vi "SettingsDialog.vi"(8 "error in (no error)":errorcluster, 11 "ProgramSettings in":refnum<class "ProgramSettings.lvclass">) -> (0 "error out":errorcluster, 3 "ProgramSettings out":refnum<class "ProgramSettings.lvclass">)   [LabVIEW 2019, in "ProgramSettings.lvclass"]
uses:
  ProgramSettings.lvclass
  ProgramSettings.lvclass/ProgramSettings.ctl
panel:
  in  "Settings":T1={"Serial Port for strømforsyning"="COM12"}
  in  "Cancel":bool
  in  "OK":bool
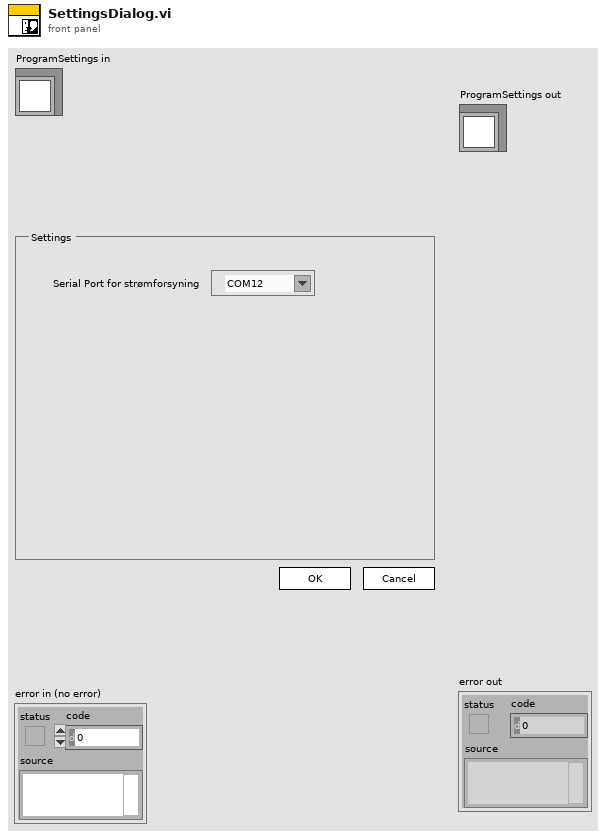
[diagram p1: front panel]
types:
  T1 = cluster{"Serial Port for strømforsyning":refnum<visa-resource-name>}
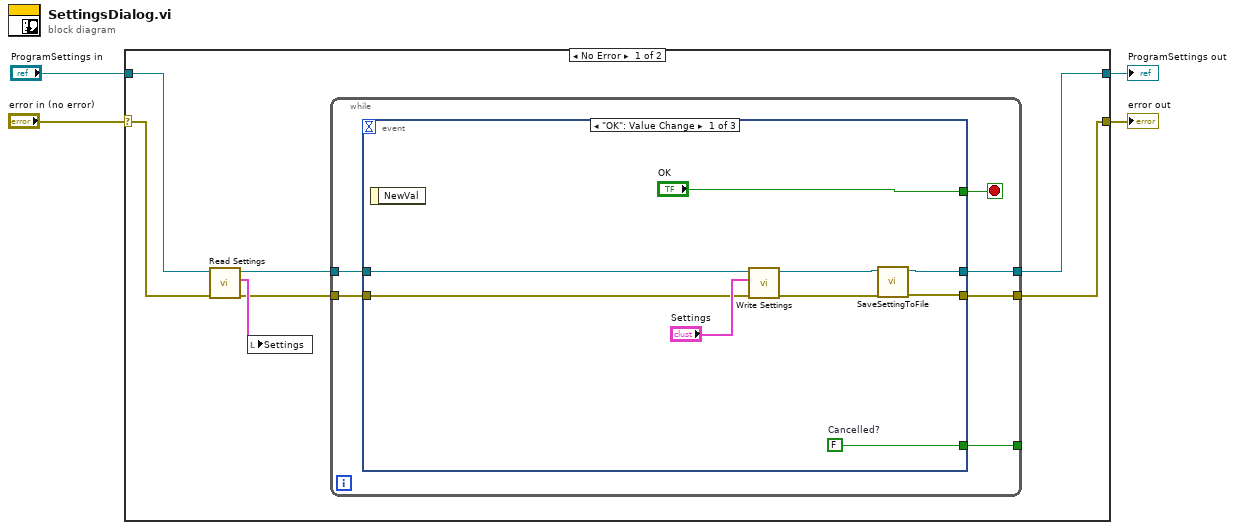
[diagram p0: block diagram]
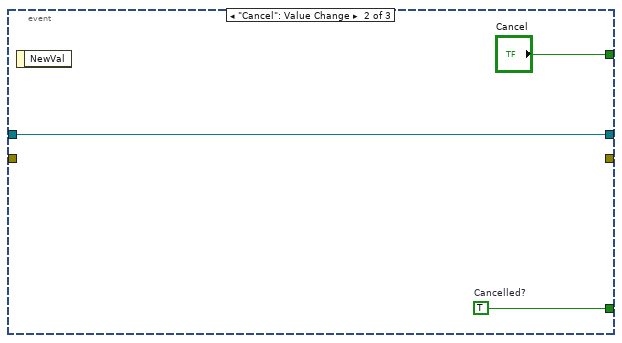
[diagram p2: hidden frame]
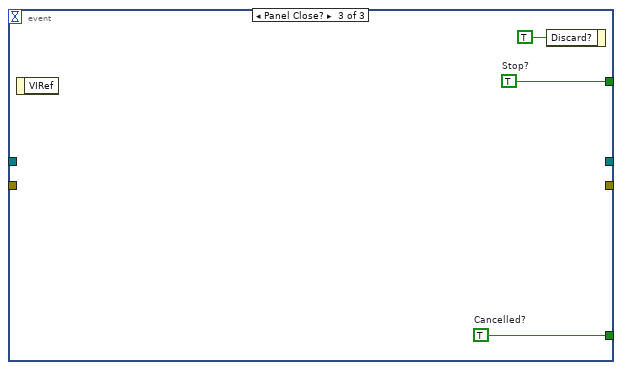
[diagram p3: hidden frame]
diagram:
  n1 = case shown="No Error" "error in (no error)" {
    selector: "error in (no error)" -> [w7 w34]
    tunnel: [w10 w34] -> w3
    tunnel: [w11 w33] -> w1
    tunnel: "ProgramSettings in" -> [w8 w33]
    frame No Error {
      n2 = call "Read Settings.vi"("error in (no error)"=w7, "ProgramSettings in"=w8) -> ("error out"=w6:errorcluster, "Settings"=w9:T1, "ProgramSettings out"=w5:refnum<class "ProgramSettings.lvclass">)  [unwired: 7 in]
      n3 = local write "Settings"(w9) -> ()
      n4 = while {
        tunnel: [w16] -> _
        tunnel: w5 -> [w15]
        tunnel: [w14] -> w11
        tunnel: w6 -> [w13]
        tunnel: [w12] -> w10
        stop <- w17 stop-if-true
        n5 = event shown="[0] \"OK\": Value Change" {
          selector: _ -> [_ _ _]
          dyn-events: _ -> [_ _ _]
          timeout: _ -> [_ _ _]
          tunnel: ["OK" "Cancel" w31] -> w17
          tunnel: [w26 w29 w30] -> w16
          tunnel: w15 -> [w23 w27 _]
          tunnel: [w20 w27 _] -> w14
          tunnel: w13 -> [w22 _ _]
          tunnel: [w18 _ _] -> w12
          event "OK": Value Change {
            w26 = FALSE  # Cancelled?
            n6 = event-data() -> ()  [unwired: 1 in, 1 out]
            n7 = call "Write Settings.vi"("error in (no error)"=w22, "Settings"="Settings", "ProgramSettings in"=w23) -> ("error out"=w19:errorcluster, "ProgramSettings out"=w21:refnum<class "ProgramSettings.lvclass">)  [unwired: 7 in]
            n8 = call "SaveSettingToFile.vi"("error in (no error)"=w19, "ProgramSettings in"=w21) -> ("error out"=w18:errorcluster, "ProgramSettings out"=w20:refnum<class "ProgramSettings.lvclass">)  [unwired: 8 in]
          }
          event "Cancel": Value Change {
            w29 = TRUE  # Cancelled?
            n9 = event-data() -> ()  [unwired: 1 in, 1 out]
          }
          event Panel Close? {
            w30 = TRUE  # Cancelled?
            w31 = TRUE  # Stop?
            n10 = event-data() -> ()  [unwired: 1 in, 1 out]
            n11 = event-data("Discard?"=TRUE) -> ()  [unwired: 1 in, 1 out]
          }
        }
      }
    }
    frame Error {
    }
  }
  "error out" <- w3
  "ProgramSettings out" <- w1
